vi "Enable Sinewave Out Value.vi"(8 "error in":errorcluster, 10 "Enable Sinewave Out":bool) -> (0 "error out":errorcluster)   [LabVIEW 2024, in "User Interface Control.lvlib"]
uses:
  User Interface Control.lvlib
  Tester Internal Communication/References - Get.vi
  Tester Internal Communication/Tester InterComm.lvlib
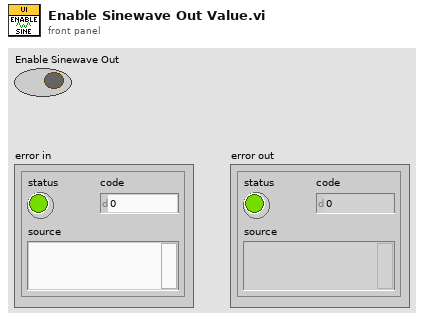
[diagram p1: front panel]
types:
  T1 = enum8{"Enabled", "Disabled", "Disabled and Grayed Out"}
  T2 = typedef "Tester InterComm.lvlib/Tester References.ctl" = cluster{"Main VI":cluster{"This VI":refnum<vi>}, "App Controls":cluster{"Test Device":refnum<vi>, "Tab Control":refnum<vi>, "STOP":refnum<vi>, "Working Mode":refnum<vi>}, "Indicators":cluster{"Messages Display":refnum<vi>, "Voltage Value":refnum<vi>, "PWM Value":refnum<vi>, "PWM Graph":refnum<vi>, "Duty Cycle":refnum<vi>, "Frequency":refnum<vi>, "Sinewave Graph":refnum<vi>, "ECU Present":refnum<vi>}, "Manufacturing Mode Controls":cluster{"Read Speed":refnum<vi>, "Voltage Out":refnum<vi>, "V Enable/Disable":refnum<vi>, "PWM Enable/Disable":refnum<vi>, "PWM Out":refnum<vi>, "Sine Enable/Disable":refnum<vi>, "Sinewave Out":refnum<vi>, "DO1":refnum<vi>, "DO2":refnum<vi>}}
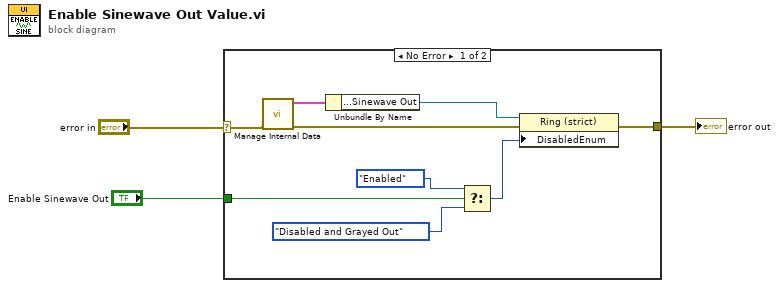
[diagram p0: block diagram]
diagram:
  n1 = case shown="No Error" "error in" {
    selector: "error in" -> [w5 w13]
    tunnel: "Enable Sinewave Out" -> [w7 _]
    tunnel: [w6 w13] -> w2
    frame No Error {
      n2 = call-poly "Manage Internal Data.vi"("error in"=w5) -> ("error out"=w11:errorcluster, "References Out"=w12:T2)  [unwired: 9 in]
      n3 = Unbundle By Name(w12) -> ("Manufacturing Mode Controls.Sinewave Out"=w4:refnum<vi>)
      n4 = Select(t=T1."Enabled" ("DisabledEnum"), s=w7, f=T1."Disabled and Grayed Out" ("DisabledEnum")) -> (s? t:f=w8:T1)
      n5 = property class="Ring (strict)"(reference=w4, error in=w11, "DisabledEnum"=w8) -> (error out=w6:errorcluster)  [unwired: 1 out]
    }
    frame Error {
    }
  }
  "error out" <- w2
